vi "Library Child Class URL.vi"(7 "Destination":path=path "", 8 "Error In":errorcluster, 11 "Name":string) -> (0 "Error Out":errorcluster, 3 "Child URL":string)   [LabVIEW 2018, in "Scripts.lvlib"]
uses:
  Scripts.lvlib
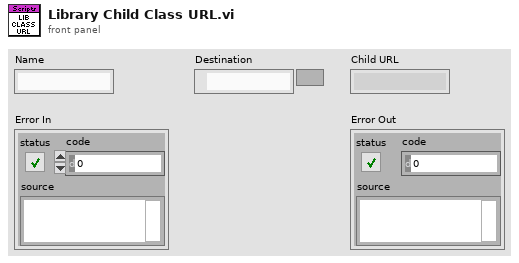
[diagram p1: front panel]
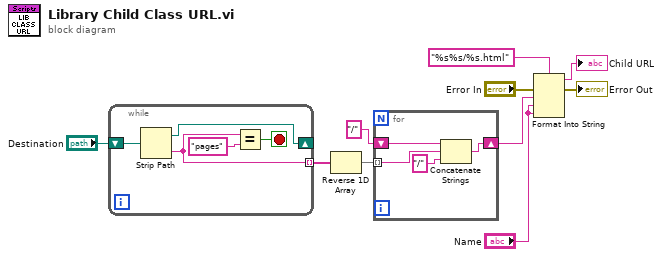
[diagram p0: block diagram]
diagram:
  n1 = while {
    shift-right: [w13] -> _
    shift-left: "Destination" -> [w14]
    tunnel: [w11] -> w1 mode=indexing
    stop <- w12 stop-if-true
    n2 = Strip Path(path=w14) -> (stripped path=w13:path, name=w11:string)
    n3 = Equal?(x=w11, y="pages") -> (x = y?=w12:bool)
  }
  n4 = Reverse 1D Array(array=w1) -> (reversed array=w4:string[])
  n5 = for {
    tunnel: w4 -> [w18] mode=indexing
    shift-right: [w16] -> w2
    shift-left: "/" -> [w19]
    n6 = Concatenate Strings(w19, w18, "/") -> (w16:string)
  }
  n7 = Format Into String(format string="%s%s/%s.html", error in="Error In", w2, "Name", "Name") -> (resulting string=→"Child URL":string, error out=→"Error Out":errorcluster)  [unwired: 1 in]
